vi "Get Script Name.vi"() -> (3 "Script Name":string)   [LabVIEW 2014]
uses:
  <vilib>/Rock Robotics/WPI/DriverStation/WPI_DriverStationRobotMode2.ctl
  <vilib>/Rock Robotics/Network Tables/SD Read Boolean.vi
  Begin/Global Variables.vi
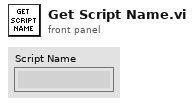
[diagram p1: front panel]
types:
  T1 = typedef "WPI_DriverStationRobotMode2.ctl" = enum16{"Autonomous Disabled", "Autonomous Enabled", "Teleop Disabled", "Teleop Enabled", "Disconnected", "Finish", "Test Disabled", "Test Enabled", "Emergency Stopped"}
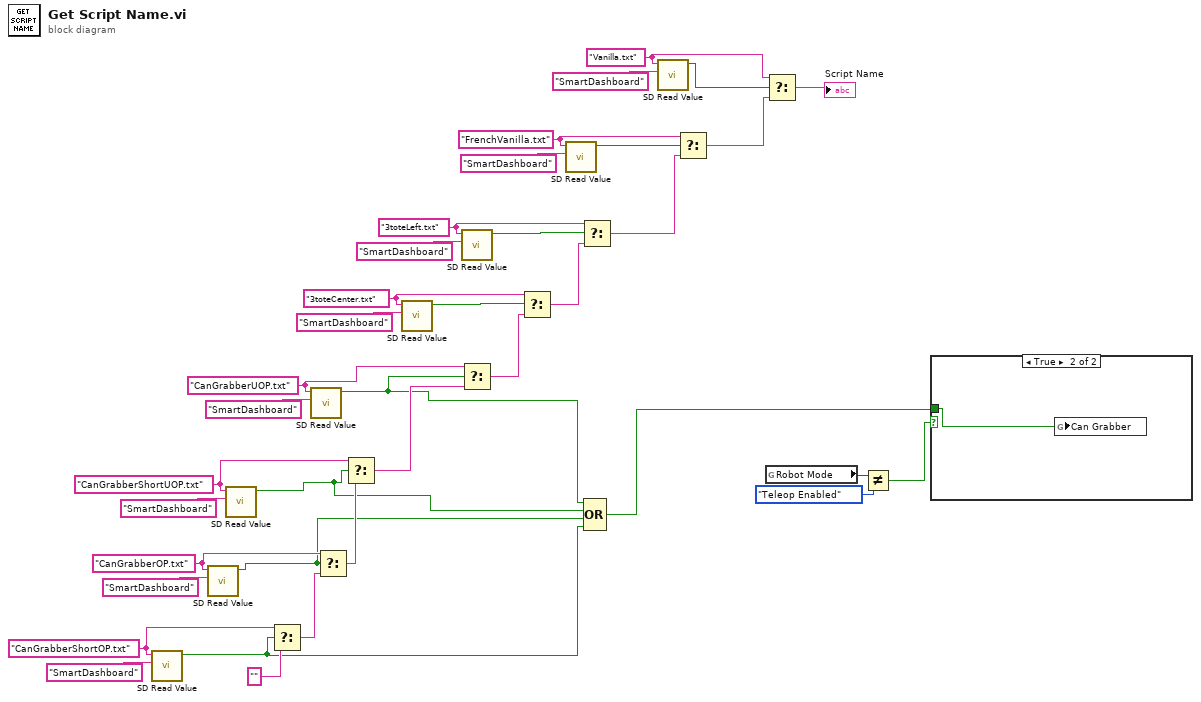
[diagram p0: block diagram]
diagram:
  w7 = "CanGrabberShortOP.txt" ("Name")
  w10 = "CanGrabberOP.txt" ("Name")
  w13 = "CanGrabberShortUOP.txt" ("Name")
  w20 = "3toteLeft.txt" ("Name")
  w24 = "CanGrabberUOP.txt" ("Name")
  w27 = "3toteCenter.txt" ("Name")
  w30 = "FrenchVanilla.txt" ("Name")
  w32 = "Vanilla.txt" ("Name")
  n1 = call-poly <vilib>:"SD Read Value.vi"("Table Prefix"="SmartDashboard", "Name"=w7) -> ("Boolean"=w1:bool)  [unwired: 7 in, 2 out]
  n2 = call-poly <vilib>:"SD Read Value.vi"("Table Prefix"="SmartDashboard", "Name"=w10) -> ("Boolean"=w3:bool)  [unwired: 7 in, 2 out]
  n3 = call-poly <vilib>:"SD Read Value.vi"("Table Prefix"="SmartDashboard", "Name"=w13) -> ("Boolean"=w4:bool)  [unwired: 7 in, 2 out]
  n4 = Select(t=w7, s=w1, f="") -> (s? t:f=w8:string)
  n5 = call-poly <vilib>:"SD Read Value.vi"("Table Prefix"="SmartDashboard", "Name"=w24) -> ("Boolean"=w5:bool)  [unwired: 7 in, 2 out]
  n6 = Select(t=w10, s=w3, f=w8) -> (s? t:f=w9:string)
  n7 = Select(t=w13, s=w4, f=w9) -> (s? t:f=w15:string)
  n8 = call-poly <vilib>:"SD Read Value.vi"("Table Prefix"="SmartDashboard", "Name"=w27) -> ("Boolean"=w28:bool)  [unwired: 7 in, 2 out]
  n9 = call-poly <vilib>:"SD Read Value.vi"("Table Prefix"="SmartDashboard", "Name"=w20) -> ("Boolean"=w19:bool)  [unwired: 7 in, 2 out]
  n10 = Select(t=w24, s=w5, f=w15) -> (s? t:f=w25:string)
  n11 = Select(t=w27, s=w28, f=w25) -> (s? t:f=w17:string)
  n12 = call-poly <vilib>:"SD Read Value.vi"("Table Prefix"="SmartDashboard", "Name"=w30) -> ("Boolean"=w29:bool)  [unwired: 7 in, 2 out]
  n13 = Select(t=w20, s=w19, f=w17) -> (s? t:f=w16:string)
  n14 = Compound Arithmetic op=OR(w5, w4, w3, w1) -> (w2:bool)
  n15 = call-poly <vilib>:"SD Read Value.vi"("Table Prefix"="SmartDashboard", "Name"=w32) -> ("Boolean"=w33:bool)  [unwired: 7 in, 2 out]
  n16 = Select(t=w30, s=w29, f=w16) -> (s? t:f=w31:string)
  n17 = global read "Global Variables.vi" "Robot Mode"() -> (w23:T1)
  n18 = Select(t=w32, s=w33, f=w31) -> (s? t:f=→"Script Name":string)
  n19 = Not Equal?(x=w23, y=WPI_DriverStationRobotMode2."Teleop Enabled") -> (x != y?=w21:bool)
  n20 = case shown="True" w21 {
    tunnel: w2 -> [_ w38]
    frame False {
    }
    frame True {
      n21 = global write "Global Variables.vi" "Can Grabber"(w38) -> ()
    }
  }
